vi "GetToolsMenuItems.vi"(0 "reference in":refnum<class "ClassDiagramGraph.lvclass">, 5 "error in (no error)":errorcluster) -> (14 "reference out":refnum<class "ClassDiagramGraph.lvclass">, 16 "ToolMenuItems":T1(array[cluster])=[{"Generate code from UML...", "createScript", "short cut out"={"include Shift key?"=FALSE, "include Ctrl key? "=FALSE, "shortcut key"=""}}, {"Reverse Engineering...", "Class Reversed Engineering", "short cut out"={"include Shift key?"=FALSE, "include Ctrl key? "=TRUE, "shortcut key"="R"}}, {"Auto Place...", "AutoPlace", "short cut out"={"include Shift key?"=FALSE, "include Ctrl key? "=FALSE, "shortcut key"=""}}, {"Synchronize all classes from code", "Synchronize All", "short cut out"={"include Shift key?"=FALSE, "include Ctrl key? "=FALSE, "shortcut key"=""}}, {"Try to straighten associations", "StraightenAssociations", "short cut out"={"include Shift key?"=FALSE, "include Ctrl key? "=TRUE, "shortcut key"="A"}}, {"Toggle auto synchronization", "ToggleSync", "short cut out"={"include Shift key?"=FALSE, "include Ctrl key? "=FALSE, "shortcut key"="F5"}}, {"-", "APP_SEPARATOR", "short cut out"={"include Shift key?"=FALSE, "include Ctrl key? "=FALSE, "shortcut key"=""}}], 19 "error out":errorcluster)   [LabVIEW 2020, in "ClassDiagramGraph.lvclass"]
uses:
  <resource>/Framework/Providers/Open_GDS/UML/ClassDiagramGraph_class/ClassDiagramGraph.lvclass
  <resource>/Framework/Providers/Open_GDS/UML/UMLEditor/UMLEditor_StoredPathes.ctl
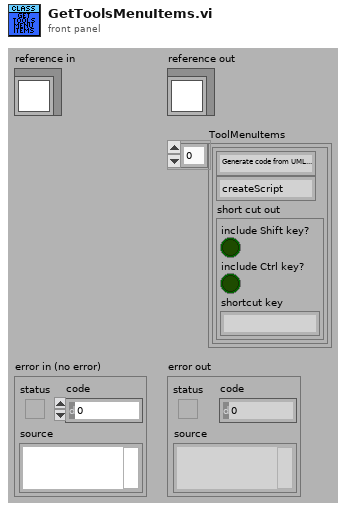
[diagram p1: front panel]
types:
  T1 = cluster{string, string, "short cut out":cluster{"include Shift key?":bool, "include Ctrl key? ":bool, "shortcut key":string}}[]
  T2 = cluster{string, string, "short cut out":cluster{"include Shift key?":bool, "include Ctrl key? ":bool, "shortcut key":string}}
  T3 = typedef "UMLEditor_StoredPathes.ctl" = enum16{"LastSearchPath", "QueuedArrayStateVI", "ClassBasePath", "ViTemplatePath", "ApplicationTemplatePath", "IniFilePath", "WizDir", "RevPlugInPath"}
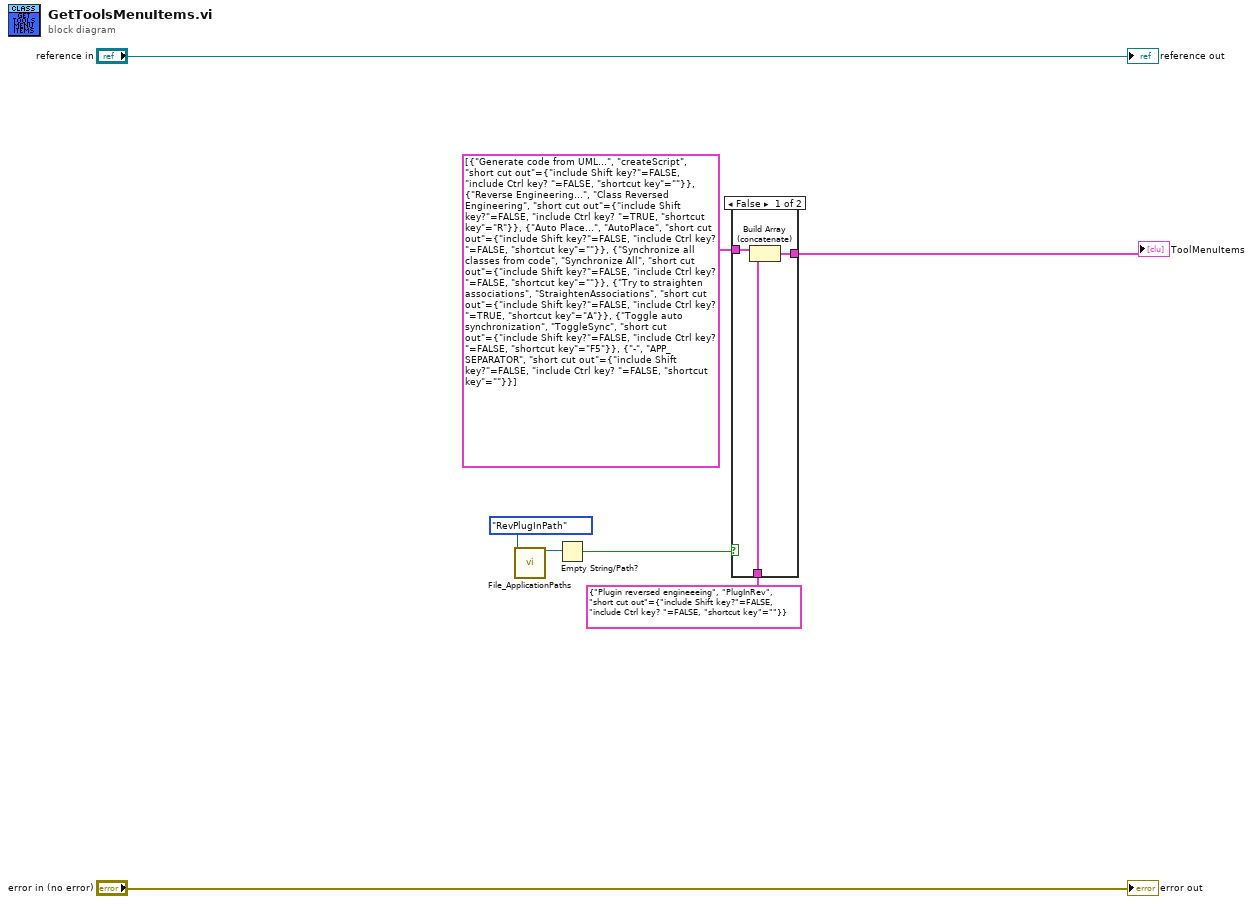
[diagram p0: block diagram]
diagram:
  n1 = call <resource>:"File_ApplicationPaths.vi"("PathName"=UMLEditor_StoredPathes."RevPlugInPath" ("UMLPathes")) -> ("Path Out"=w5:path)  [unwired: 3 in, 15 out]
  n2 = Empty String/Path?(string/path=w5) -> (empty?=w4:bool)
  n3 = case shown="False" w4 {
    tunnel: [w10 w12] -> w1
    tunnel: T1 [{"Generate code from UML...", "createScript", "short cut out"={"include Shift key?"=FALSE, "include Ctrl key? "=FALSE, "shortcut key"=""}}, {"Reverse Engineering...", "Class Reversed Engineering", "short cut out"={"include Shift key?"=FALSE, "include Ctrl key? "=TRUE, "shortcut key"="R"}}, {"Auto Place...", "AutoPlace", "short cut out"={"include Shift key?"=FALSE, "include Ctrl key? "=FALSE, "shortcut key"=""}}, {"Synchronize all classes from code", "Synchronize All", "short cut out"={"include Shift key?"=FALSE, "include Ctrl key? "=FALSE, "shortcut key"=""}}, {"Try to straighten associations", "StraightenAssociations", "short cut out"={"include Shift key?"=FALSE, "include Ctrl key? "=TRUE, "shortcut key"="A"}}, {"Toggle auto synchronization", "ToggleSync", "short cut out"={"include Shift key?"=FALSE, "include Ctrl key? "=FALSE, "shortcut key"="F5"}}, {"-", "APP_SEPARATOR", "short cut out"={"include Shift key?"=FALSE, "include Ctrl key? "=FALSE, "shortcut key"=""}}] -> [w11 w12]
    tunnel: T2 {"Plugin reversed engineeeing", "PlugInRev", "short cut out"={"include Shift key?"=FALSE, "include Ctrl key? "=FALSE, "shortcut key"=""}} -> [w9 _]
    frame False {
      n4 = Build Array (concatenate)(w11, w9) -> (w10:T1)
    }
    frame True {
    }
  }
  "ToolMenuItems" <- w1
  "error out" <- "error in (no error)"
  "reference out" <- "reference in"
